vi "asset.get.vi"(8 "error in":errorcluster, 10 "Asset RID":string, 11 "Nominal Client in":refnum<class "Nominal Client.lvclass">) -> (0 "error out":errorcluster, 2 "Asset":refnum<class "asset.lvclass">, 3 "Nominal Client out":refnum<class "Nominal Client.lvclass">)   [LabVIEW 2020, in "Nominal Client.lvclass"]
doc: "Triggers an ingest job, allowing either creating a new dataset or uploading to an existing one. This endpoint is meant to supersede all other ingestion endpoints as their functionality gets migrated to this one."
uses:
  Nominal Client.lvclass
  asset/asset.lvclass
  Nominal Client.lvclass/Nominal Client.ctl
  nominal types/workspace/rid.get.vi
  c20a9d0c-990e-4b00-9818-b2ddac785778.vi
  trace.payload_received.vi
  error.vi
  trace.payload_sent.vi
  create.authorization_header.vi
  trace.generate.vi
  trace.calling_method.vi
  error.vi/859f8e04-e495-489b-b5b4-7ac163f56130.vi
  <vilib>/AdvancedString/1D String Array to Delimited String.vi
  <vilib>/JDP Science/JDP Science Common Utilities/Trim Whitespace__JDP.vi
  api_token.get.vi
  <vilib>/JDP Science/JSONtext/Variant to JSON Text.vi
  <vilib>/Utility/libraryn.llb/Get File Extension.vi
  log_file.write.vi
  <vilib>/Utility/error.llb/Error Cluster From Error Code.vi
  <vilib>/JDP Science/JSONtext/JSON text to Variant.vi
  <vilib>/JDP Science/JSONtext/LVClass Serializer/JSONtext LVClass Serializer.lvclass
  <vilib>/addons/_JKI.lib/REST Client/classes/Response Headers/Response Headers.lvclass
  <vilib>/addons/_JKI.lib/REST Client/classes/REST Client/REST Client.lvclass
  <vilib>/JDP Science/JSONtext/JSONtext.lvlib
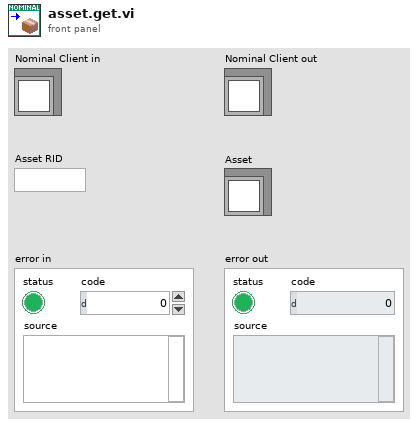
[diagram p1: front panel]
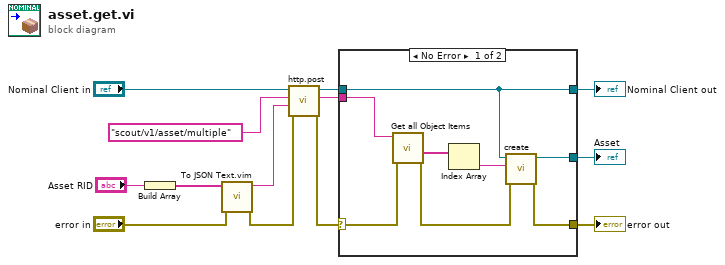
[diagram p0: block diagram]
diagram:
  n1 = Build Array("Asset RID") -> (w2:string[])
  n2 = call "To JSON Text.vim"("error in (no error)"="error in", "Anything"=w2) -> ("error out"=w4:errorcluster, "<JSON>"=w5:string)  [unwired: 8 in]
  n3 = call "http.post.vi"("error in"=w4, "Request body"=w5, "Path"="scout/v1/asset/multiple", "Nominal Client in"="Nominal Client in") -> ("error out"=w8:errorcluster, "Response"=w12:string, "Nominal Client out"=w10:refnum<class "Nominal Client.lvclass">)  [unwired: 4 in, 1 out]
  n4 = case shown="No Error" w8 {
    selector: w8 -> [w14 w23]
    tunnel: w12 -> [w20 _]
    tunnel: w10 -> [w15 w22]
    tunnel: [w15 w22] -> w9
    tunnel: [w21 w23] -> w7
    tunnel: [w16 _] -> w1
    frame No Error {
      n5 = call <vilib>:"Get all Object Items.vi"("error in (no error)"=w14, "JSON"=w20) -> ("error out"=w19:errorcluster, "<JSON>"=w18:string[])  [unwired: 6 in, 2 out]
      n6 = Index Array(array=w18) -> (element=w17:string)  [unwired: 1 in]
      n7 = call "create.vi"("error in"=w19, "asset"=w17, "Nominal Client"=w15) -> ("error out"=w21:errorcluster, "asset"=w16:refnum<class "asset.lvclass">)  [unwired: 7 in]
    }
    frame Error {
    }
  }
  "Nominal Client out" <- w9
  "error out" <- w7
  "Asset" <- w1
